vi "Initialize Simulated Starter Kit 2.0.vi"(8 "error in (no error)":errorcluster, 11 "robot ID":string="Starter Kit 2.0_R0") -> (0 "error out":errorcluster, 3 "simulated starter kit host 2.0 out":refnum<class "NI_Robotics_Starter Kit Host_Sim_2.0.lvclass">)   [LabVIEW 2017, in "NI_Robotics_Starter Kit Host_Sim_2.0.lvclass"]
doc: "Begins a communication session for a simulated Starter Kit 2.0 robot."
uses:
  <vilib>/robotics/Starter Kit/2.0/Sim Host Interface/NI_Robotics_Starter Kit Host_Sim_2.0.lvclass
  c:/Program Files (x86)/National Instruments/LabVIEW 2017/vi.lib/robotics/Starter Kit/Sim Host Interface/NI_Robotics_Starter Kit Host_Sim.lvclass
  c:/Program Files (x86)/National Instruments/LabVIEW 2017/vi.lib/robotics/Starter Kit/Host Interface/NI_Robotics_Starter Kit Host.lvclass
  <vilib>/robotics/Starter Kit/Host Interface/NI_Robotics_Starter Kit Host.lvclass/NI_Robotics_Starter Kit Host.ctl
  <vilib>/robotics/Starter Kit/Sim Host Interface/NI_Robotics_Starter Kit Host_Sim.lvclass
  <vilib>/robotics/Starter Kit/Host Interface/NI_Robotics_Starter Kit Host.lvclass
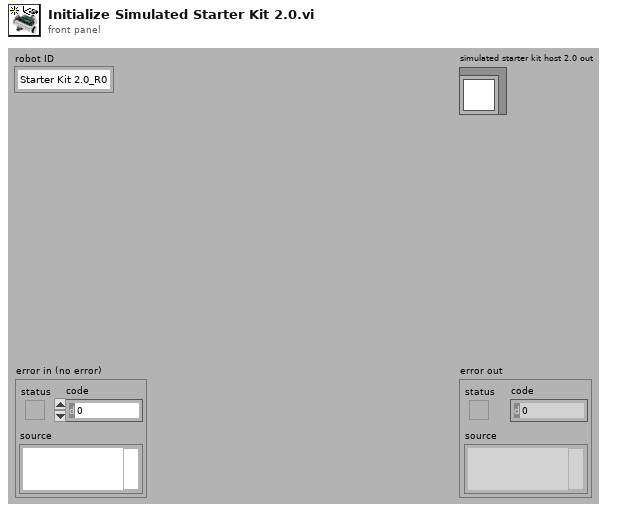
[diagram p1: front panel]
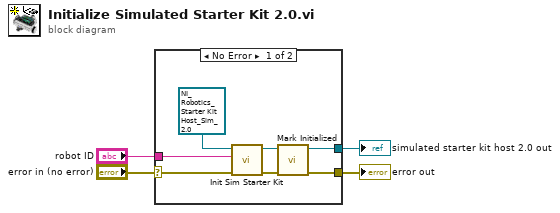
[diagram p0: block diagram]
diagram:
  n1 = case shown="No Error" "error in (no error)" {
    selector: "error in (no error)" -> [w11 w12]
    tunnel: [w6 w12] -> w2
    tunnel: [w8 _] -> w3
    tunnel: "robot ID" -> [w5 _]
    frame No Error {
      n2 = call <vilib>:"Init Sim Starter Kit.vi"("error in (no error)"=w11, "robot ID"=w5, "sim starter hit host in"=refnum<class "NI_Robotics_Starter Kit Host_Sim_2.0.lvclass"> refnum ("NI_Robotics_Starter Kit Host_Sim_2.0 out")) -> ("error out"=w7:errorcluster, "sim starter hit host out"=w9:refnum<class "NI_Robotics_Starter Kit Host_Sim_2.0.lvclass">)  [unwired: 7 in]
      n3 = call <vilib>:"Mark Initialized.vi"("error in (no error)"=w7, "starter kit host in"=w9) -> ("error out"=w6:errorcluster, "starter kit host out"=w8:refnum<class "NI_Robotics_Starter Kit Host_Sim_2.0.lvclass">)  [unwired: 8 in]
    }
    frame Error {
    }
  }
  "error out" <- w2
  "simulated starter kit host 2.0 out" <- w3
